vi "AlliGator Add New Gate to Dataset Images.vi"(7 "Buffer Image available?":bool, 8 "error in (no error)":errorcluster, 9 "Current Gate":i32, 10 "New Gate Image Refnum":T1, 11 "Dataset Images in":T2) -> (0 "error out":errorcluster, 1 "Current Gate (dup)":i32, 3 "Dataset Images out":T2)   [LabVIEW 2021, in "AlliGator Files.lvlib"]
doc: "Adds new gate image to dataset image structure."
uses:
  AlliGator Files.lvlib
  AlliGator Gate Image Set.ctl
  <vilib>/vision/Image Controls.llb/IMAQ Image.ctl
panel:
  # "see the AlliGator License on the block diagram (Ctrl+E or Window:Show Block Diagram)"
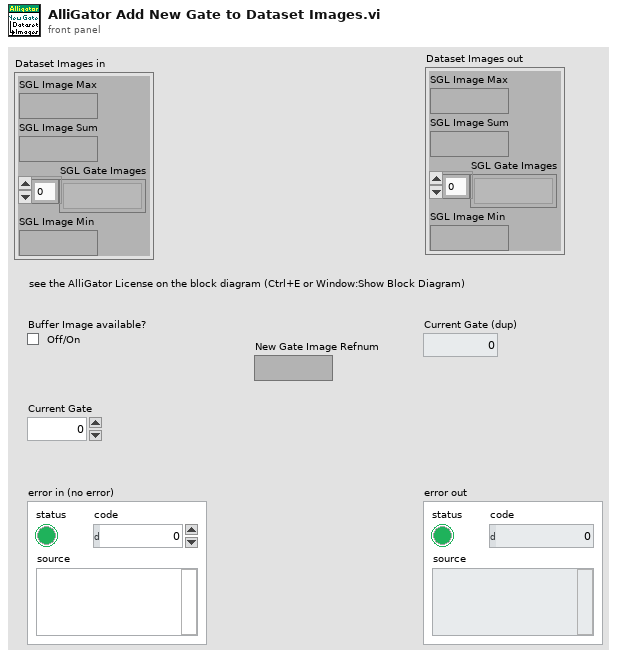
[diagram p1: front panel]
types:
  T1 = typedef "IMAQ Image.ctl" = refnum<image>
  T2 = typedef "AlliGator Files.lvlib/AlliGator Gate Image Set.ctl" = cluster{"SGL Image Max":T1, "SGL Image Sum":T1, "SGL Gate Images":T1[], "SGL Image Min":T1}
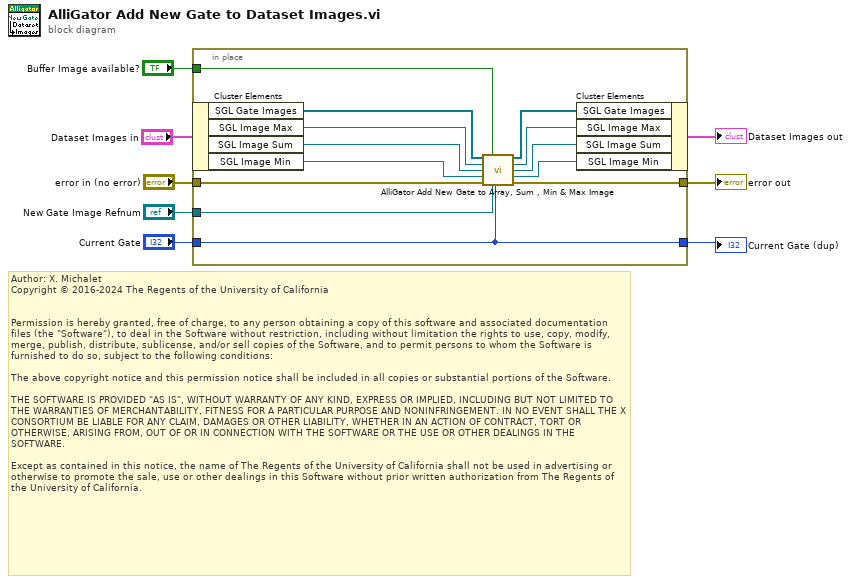
[diagram p0: block diagram]
diagram:
  # "Author: X. Michalet\nCopyright © 2016-2024 The Regents of the University of California\n \n\nPermission is hereby granted, free of charge, to any person obtaining a copy of this software and associated documentation files (the \"Software\"), to deal in the Software without restriction, including without limitation the rights to use, copy, modify, merge, publish, distribute, sublicense, and/or sell copies of the Software, and to permit persons to whom the Software is furnished to do so, subject to the following conditions:\n\nThe above copyright notice and this permission notice shall be included in all copies or substantial portions of the Software.\n\nTHE SOFTWARE IS PROVIDED \"AS IS\", WITHOUT WARRANTY OF ANY KIND, EXPRESS OR IMPLIED, INCLUDING BUT NOT LIMITED TO THE WARRANTIES OF MERCHANTABILITY, FITNESS FOR A PARTICULAR PURPOSE AND NONINFRINGEMENT. IN NO EVENT SHALL THE X CONSORTIUM BE LIABLE FOR ANY CLAIM, DAMAGES OR OTHER LIABILITY, WHETHER IN AN ACTION OF CONTRACT, TORT OR OTHERWISE, ARISING FROM, OUT OF OR IN CONNECTION WITH THE SOFTWARE OR THE USE OR OTHER DEALINGS IN THE SOFTWARE.\n\nExcept as contained in this notice, the name of The Regents of the University of California shall not be used in advertising or otherwise to promote the sale, use or other dealings in this Software without prior written authorization from The Regents of the University of California."
  n1 = in-place {
    in-place-border: "Buffer Image available?" -> [w21]
    in-place-border: "error in (no error)" -> [w20]
    in-place-border: "New Gate Image Refnum" -> [w19]
    in-place-border: [w18] -> w5
    in-place-border: "Current Gate" -> [w17]
    in-place-border: [w17] -> w3
    n2 = in-place-cluster #1("Dataset Images in") -> ("SGL Gate Images"=w16:T1[], "SGL Image Max"=w14:T1, "SGL Image Sum"=w12:T1, "SGL Image Min"=w10:T1)
    n3 = call "AlliGator Add New Gate to Array, Sum , Min & Max Image.vi"("SGL Gate Images in"=w16, "Buffer Image Available"=w21, "SGL Image Max in"=w14, "SGL Image Sum in"=w12, "SGL Image Min in"=w10, "error in (no error)"=w20, "Gate Image"=w19, "Current Gate"=w17) -> ("SGL Gate Images out"=w15:T1[], "SGL Image Max out"=w13:T1, "SGL Image Sum out"=w11:T1, "SGL Image Min out"=w9:T1, "error out"=w18:errorcluster)  [unwired: 3 in]
    n4 = in-place-cluster #1("SGL Gate Images"=w15, "SGL Image Max"=w13, "SGL Image Sum"=w11, "SGL Image Min"=w9) -> (→"Dataset Images out":T2)
  }
  "Current Gate (dup)" <- w3
  "error out" <- w5
